vi "Mandelbrot_LabVIEW.vi"(7 "Max_iter":i32=4000, 8 "Zoom":dbl=5e-11, 9 "y":dbl=0.13182590420533, 10 "x":dbl=-0.743643887037151, 11 "Resolution":i32=1000) -> (0 "Exec Time":dbl=3.6367448000000877, 3 "Mandelbrot Intensity Graph":dbl[][](graph))   [LabVIEW 2020]
uses:
  <vilib>/Analysis/NI_AALBase.lvlib
  <vilib>/Analysis/1siggen.llb/Ramp Pattern by Samples.vi
  250ad98c-c819-4240-bb72-613057cdb05b.vi
  8fc4144a-0758-458b-88ac-401a6681cd74.vi
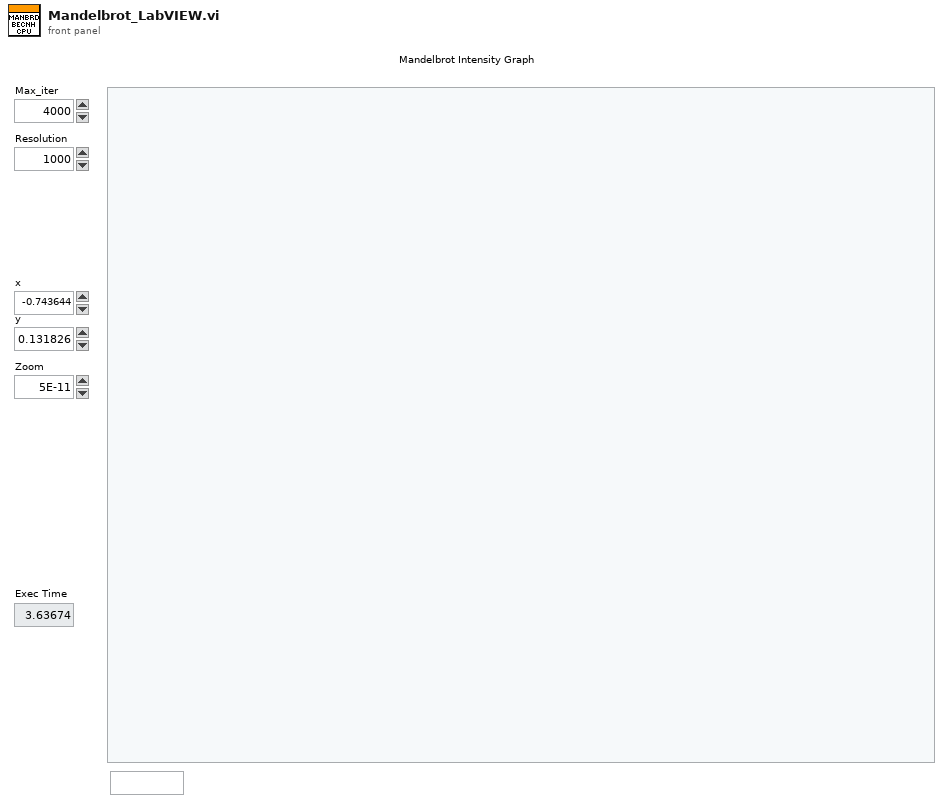
[diagram p1: front panel]
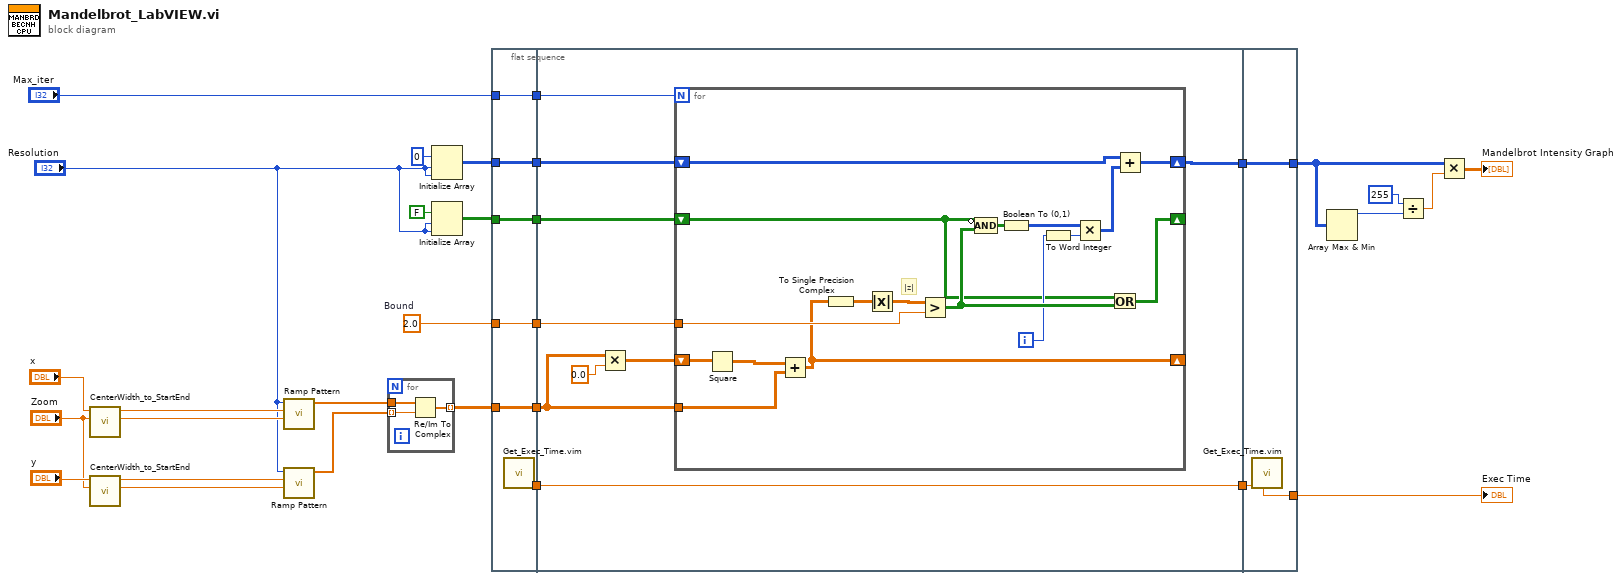
[diagram p0: block diagram]
diagram:
  w16 = sgl 2.0  # Bound
  n1 = call "CenterWidth_to_StartEnd.vi"("width"="Zoom", "Center"="x") -> ("Start"=w22:dbl, "End"=w23:dbl)  [unwired: 8 in]
  n2 = call "CenterWidth_to_StartEnd.vi"("width"="Zoom", "Center"="y") -> ("Start"=w18:dbl, "End"=w19:dbl)  [unwired: 8 in]
  n3 = call-poly <vilib>:"Ramp Pattern.vi"("start"=w22, "end"=w23, "samples"="Resolution") -> ("Ramp Pattern"=w21:dbl[])  [unwired: 7 in, 1 out]
  n4 = call-poly <vilib>:"Ramp Pattern.vi"("start"=w18, "end"=w19, "samples"="Resolution") -> ("Ramp Pattern"=w20:dbl[])  [unwired: 7 in, 1 out]
  n5 = for {
    tunnel: w20 -> [w33] mode=indexing
    tunnel: w21 -> [w34]
    tunnel: [w32] -> w17 mode=indexing
    n6 = Re/Im To Complex(1:w33, 2:w34) -> (0:w32:cdb[])
  }
  n7 = Initialize Array(i16 0 ("element"), "Resolution", "Resolution") -> (w14:i16[][])
  n8 = Initialize Array(FALSE, "Resolution", "Resolution") -> (w12:bool[][])
  n9 = flat-sequence {
    tunnel: w17 -> [w38]
    tunnel: w12 -> [w39]
    tunnel: "Max_iter" -> [w40]
    tunnel: [w40] -> w31
    tunnel: [w39] -> w30
    tunnel: [w38] -> w29
    tunnel: [w37] -> w28
    tunnel: [w36] -> w27
    tunnel: w14 -> [w36]
    tunnel: [w35] -> w26
    tunnel: w16 -> [w35]
    tunnel: w31 -> [w49]
    tunnel: w30 -> [w41]
    tunnel: w29 -> [w48]
    tunnel: [w45] -> w25
    tunnel: w28 -> [w45]
    tunnel: w27 -> [w42]
    tunnel: [w43] -> w24
    tunnel: w26 -> [w44]
    tunnel: w25 -> [w69]
    tunnel: [w68] -> w11
    tunnel: [w67] -> w2
    tunnel: w24 -> [w67]
    frame #0 {
      n10 = call "Get_Exec_Time.vim"() -> ("T(n)"=w37:dbl)  [unwired: 7 in, 2 out]
    }
    frame #1 {
      n11 = Multiply(x=w48, y=sgl 0.0 ("start")) -> (x*y=w47:cdb[][])
      n12 = for {
        N: w49 -> [_]
        shift-right: [w55] -> _
        shift-left: w47 -> [w56]
        tunnel: w48 -> [w63]
        shift-right: [w66] -> w43
        shift-left: w42 -> [w59]
        tunnel: w44 -> [w64]
        shift-right: [w65] -> _
        shift-left: w41 -> [w51]
        i -> [w57]
        # "|z|"
        n13 = Square(x=w56) -> (x^2=w52:cdb[][])
        n14 = Add(x=w52, y=w63) -> (x+y=w55:cdb[][])
        n15 = To Single Precision Complex(1:w55) -> (0:w53:csg[][])
        n16 = Absolute Value(x=w53) -> (abs(x)=w54:sgl[][])
        n17 = Greater?(x=w54, y=w64) -> (0:w62:bool[][])
        n18 = Compound Arithmetic op=AND(invert w51, w62) -> (w61:bool[][])
        n19 = Boolean To (0,1)(Boolean=w61) -> (0, 1=w58:i16[][])
        n20 = To Word Integer(number=w57) -> (16bit integer=w50:i16)
        n21 = Multiply(x=w58, y=w50) -> (x*y=w60:i16[][])
        n22 = Or(x=w51, y=w62) -> (x .or. y?=w65:bool[][])
        n23 = Add(x=w59, y=w60) -> (x+y=w66:i16[][])
      }
    }
    frame #2 {
      n24 = call "Get_Exec_Time.vim"("T(n-1)"=w69) -> ("dT"=w68:dbl)  [unwired: 6 in, 2 out]
    }
  }
  n25 = Array Max & Min(array=w2) -> (max value=w3:i16)  [unwired: 3 out]
  n26 = Divide(x=i16 255, y=w3) -> (x/y=w5:dbl)
  n27 = Multiply(x=w2, y=w5) -> (x*y=→"Mandelbrot Intensity Graph":dbl[][])
  "Exec Time" <- w11
